vi "Set Strings from Ref.vi"(8 "error in (no error)":errorcluster, 9 "Language Index (0)":i32, 10 "GObj Refnum":refnum<vi>, 11 "GraphChart in":refnum<class "GraphChart.lvclass">) -> (0 "error out":errorcluster, 3 "GraphChart out":refnum<class "GraphChart.lvclass">)   [LabVIEW 2013, in "SET Project Data.lvlib" / "GraphChart.lvclass"]
uses:
  GraphChart.lvclass
  Control/Control.lvclass
  GObject/GObject.lvclass
  SET Project Data.lvlib
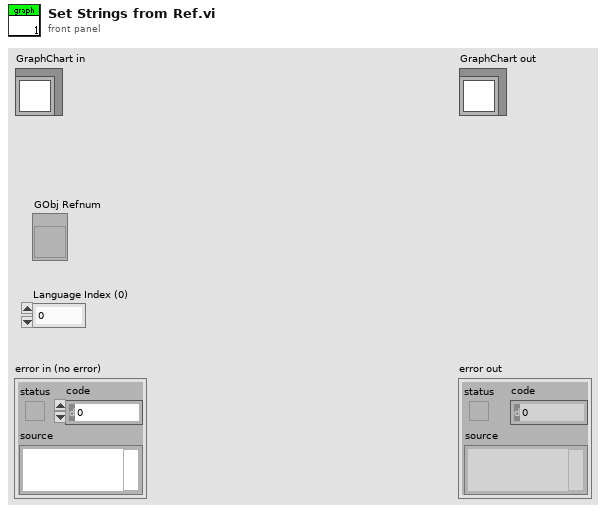
[diagram p1: front panel]
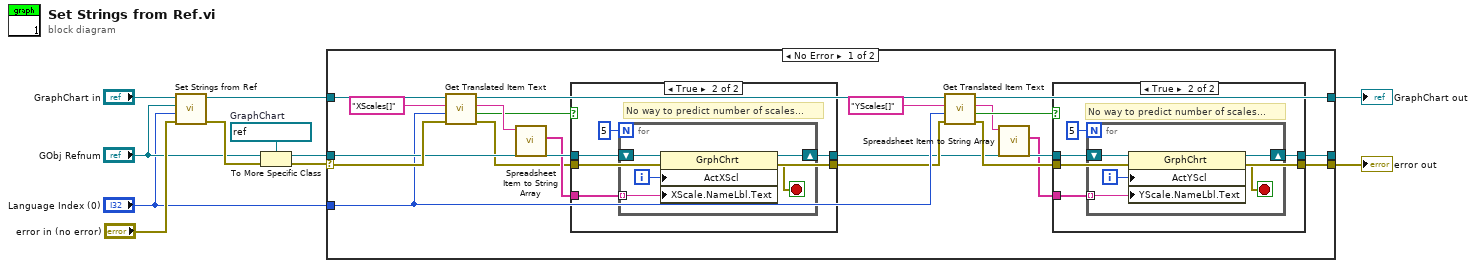
[diagram p0: block diagram]
diagram:
  w7 = refnum<vi> refnum  # GraphChart
  n1 = call-parent "Set Strings from Ref.vi"("error in (no error)"="error in (no error)", "Language Index (0)"="Language Index (0)", "GObj Refnum"="GObj Refnum", "Control in"="GraphChart in") -> ("error out"=w5:errorcluster, "Control out"=w6:refnum<class "GraphChart.lvclass">)  [unwired: 6 in]
  n2 = To More Specific Class(target class=w7, reference="GObj Refnum", error in=w5) -> (specific class reference=w9:refnum<vi>, error out=w8:errorcluster)
  n3 = case shown="No Error" w8 {
    selector: w8 -> [w28 w57]
    tunnel: w9 -> [w26 w56]
    tunnel: w6 -> [w30 w58]
    tunnel: "Language Index (0)" -> [w20 _]
    tunnel: [w16 w58] -> w2
    tunnel: [w13 w57] -> w1
    tunnel: [w12 w56] -> _
    frame No Error {
      n4 = call "Get Translated Item Text.vi"("error in (no error)"=w28, "LangIndex (0)"=w20, "ItemName"="XScales[]", "GObject in"=w30) -> ("error out"=w24:errorcluster, "Found?"=w27:bool, "Translated Text (ASCII)"=w29:string, "GObject out"=w22:refnum<class "GraphChart.lvclass">)  [unwired: 4 in]
      n5 = call "Spreadsheet Item to String Array.vi"("Spreadsheet Item (ASCII)"=w29) -> ("Strings [] (ASCII)"=w25:string[])  [unwired: 10 in]
      n6 = case shown="True" w27 {
        tunnel: w26 -> [w44 w46]
        tunnel: w25 -> [_ w50]
        tunnel: w24 -> [w45 w47]
        tunnel: [w45 w47] -> w19
        tunnel: [w44 w48] -> w17
        frame False {
        }
        frame True {
          # "No way to predict number of scales..."
          n7 = for {
            N: 5 -> [_]
            tunnel: w50 -> [w53] mode=indexing
            shift-right: [w52] -> w48
            shift-left: w46 -> [w55]
            i -> [w54]
            stop <- w51 stop-if-true
            n8 = property class="GrphChrt"(reference=w55, "ActXScl"=w54, "XScale.NameLbl.Text"=w53) -> (reference out=w52:refnum<vi>, error out=w51:errorcluster)  [unwired: 1 in]
          }
        }
      }
      n9 = call "Get Translated Item Text.vi"("error in (no error)"=w19, "LangIndex (0)"=w20, "ItemName"="YScales[]", "GObject in"=w22) -> ("error out"=w18:errorcluster, "Found?"=w21:bool, "Translated Text (ASCII)"=w15:string, "GObject out"=w16:refnum<class "GraphChart.lvclass">)  [unwired: 4 in]
      n10 = call "Spreadsheet Item to String Array.vi"("Spreadsheet Item (ASCII)"=w15) -> ("Strings [] (ASCII)"=w14:string[])  [unwired: 10 in]
      n11 = case shown="True" w21 {
        tunnel: w17 -> [w32 w38]
        tunnel: w14 -> [_ w37]
        tunnel: w18 -> [w33 w34]
        tunnel: [w33 w34] -> w13
        tunnel: [w32 w35] -> w12
        frame False {
        }
        frame True {
          # "No way to predict number of scales..."
          n12 = for {
            N: 5 -> [_]
            tunnel: w37 -> [w41] mode=indexing
            shift-right: [w40] -> w35
            shift-left: w38 -> [w43]
            i -> [w42]
            stop <- w39 stop-if-true
            n13 = property class="GrphChrt"(reference=w43, "ActYScl"=w42, "YScale.NameLbl.Text"=w41) -> (reference out=w40:refnum<vi>, error out=w39:errorcluster)  [unwired: 1 in]
          }
        }
      }
    }
    frame Error {
    }
  }
  "error out" <- w1
  "GraphChart out" <- w2
